vi "Chirp signal generator.vi"(2 "Time per integer frequency [sec]":i32=2, 4 "Append deceleration profile":bool=TRUE, 5 "Amplitude [deg]":dbl, 6 "Error In":errorcluster, 7 "Signal sampling period [ms]":i32=5 step=1, 8 "End frequency \n[Hz, cycles/sec]":i32=10 step=1, 9 "Start frequency \n[Hz, cycles/sec]":i32=1 step=1) -> (0 "error out":errorcluster, 1 "Duration of full profile [sec]":i32, 3 "Full chirp profile":dbl[](array[numeric]))   [LabVIEW 2018]
uses:
  <vilib>/Analysis/NI_AALBase.lvlib
panel:
  out "Sampled deceleration profile":dbl[](array[numeric])
  out "Deceleration profile":cluster{i32, dbl[unit], "Chirp Pattern":dbl[]}(graph)
  out "Samples in full profile":i32
  out "Full chirp profile":T1(graph)={0.0, 0.01, "arbitrary wave"=[]}
  out "Sampled chirp signal":dbl[](array[numeric])
  out "Number of samples in chirp":i32
  out "Chirp duration [sec]":i32
  out "Signal sampling rate \n[Hz, samples/sec]":dbl=100.0 step=1.0 format="%#.3g"
  out "Chirp signal":T2(graph)
  # "INPUTS"
  # "OUTPUTS"
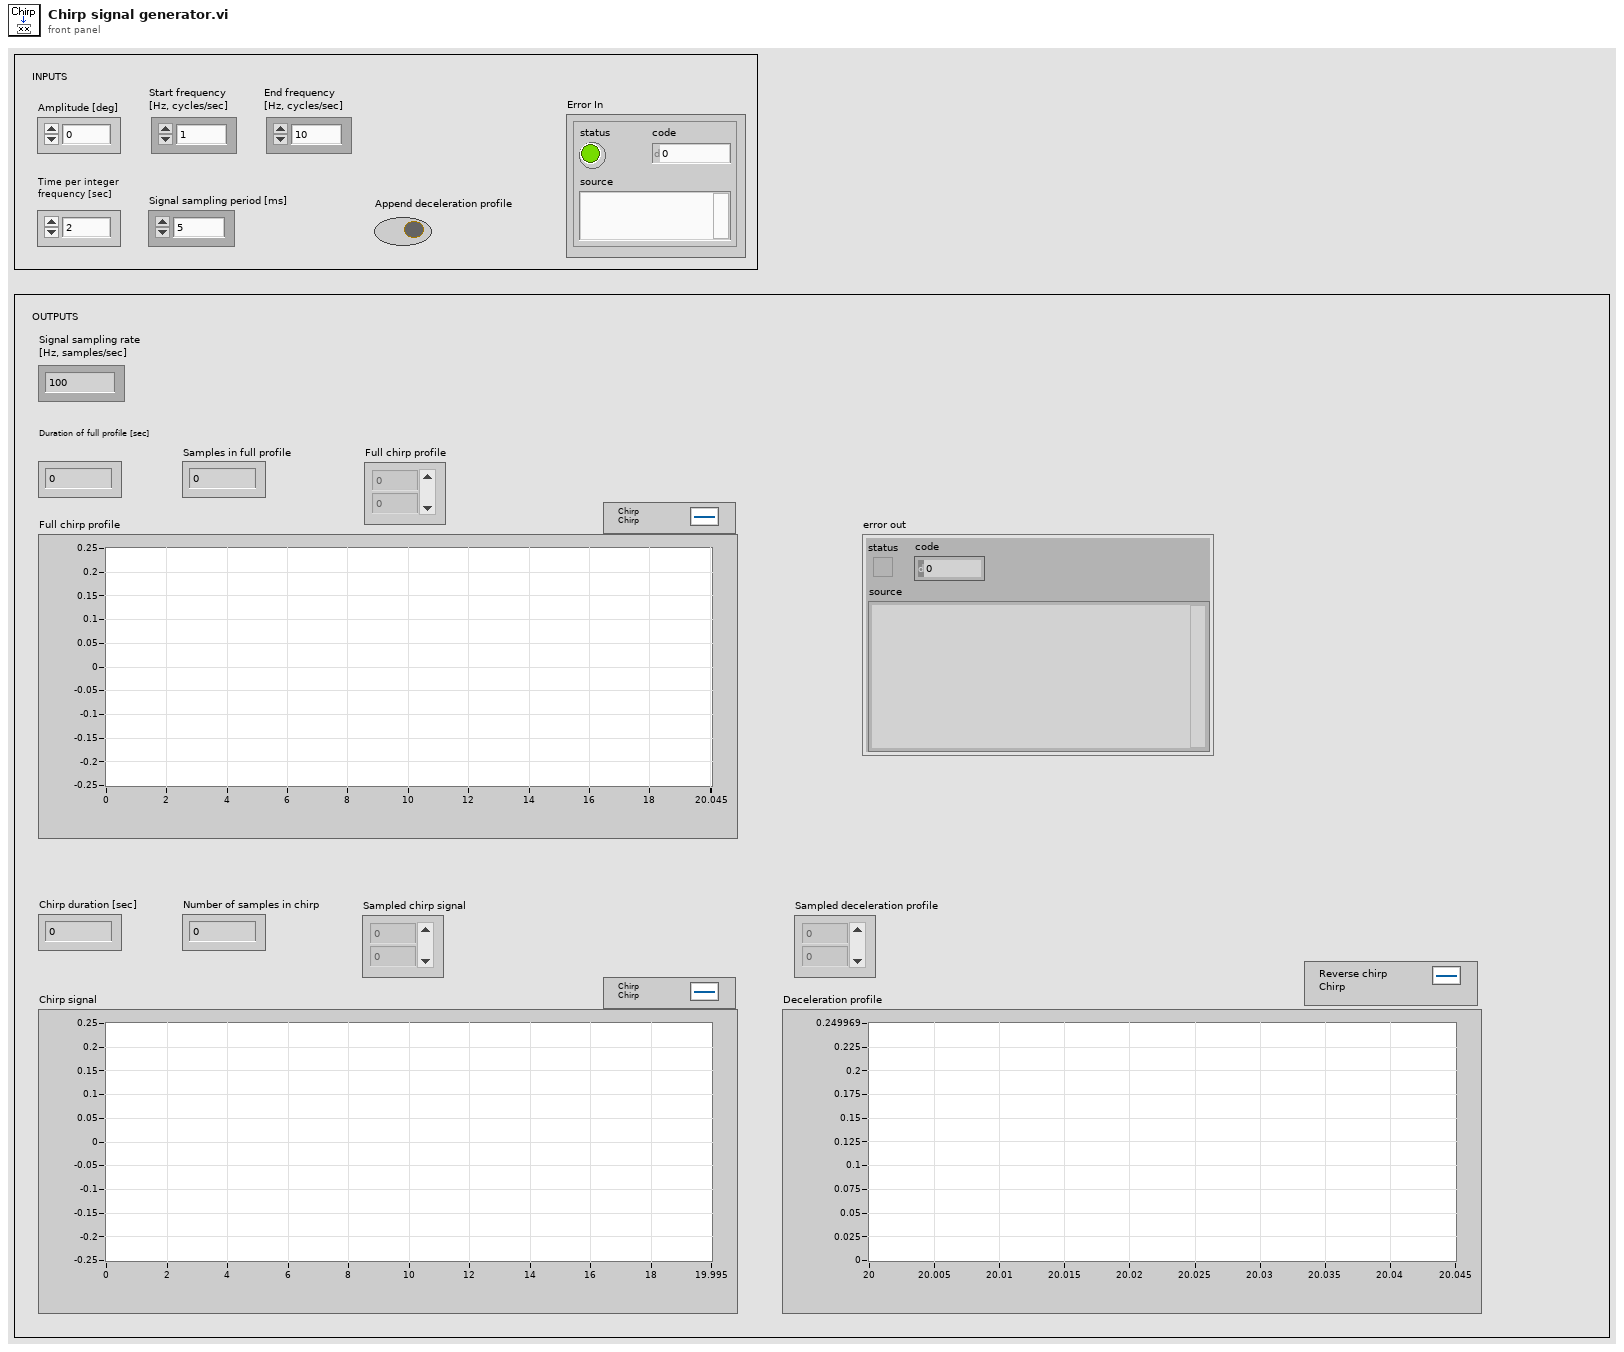
[diagram p1: front panel]
types:
  T1 = cluster{dbl[unit], dbl[unit], "arbitrary wave":dbl[]}
  T2 = cluster{dbl[unit], dbl[unit], "Chirp Pattern":dbl[]}
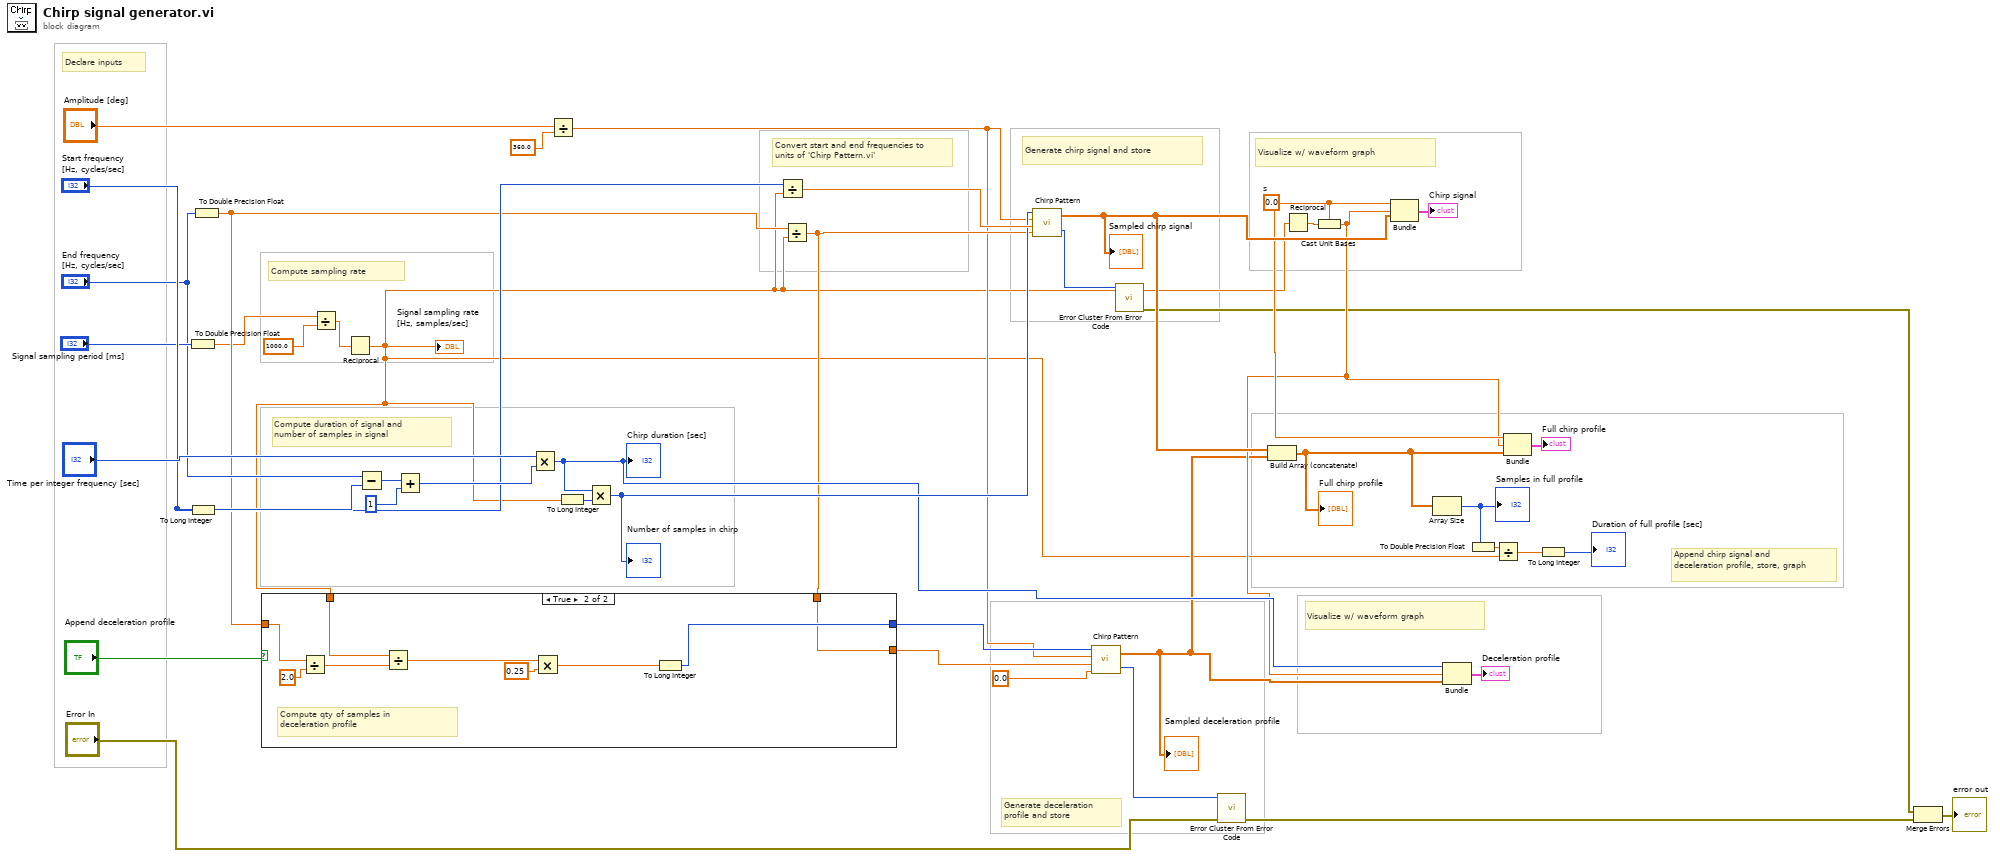
[diagram p0: block diagram]
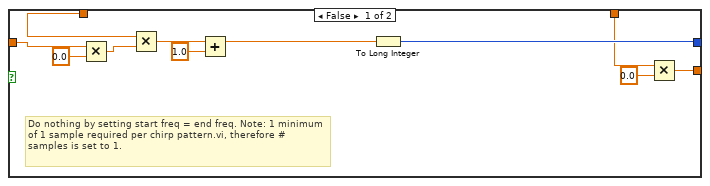
[diagram p2: hidden frame]
diagram:
  w26 = dbl[unit] 0.0  # s
  # "Generate deceleration profile and store"
  # "Visualize w/ waveform graph"
  # "Append chirp signal and deceleration profile, store, graph"
  # "Generate chirp signal and store"
  # "Visualize w/ waveform graph"
  # "Declare inputs"
  # "Convert start and end frequencies to units of 'Chirp Pattern.vi'"
  # "Compute sampling rate"
  # "Compute duration of signal and number of samples in signal"
  n1 = To Double Precision Float(number="Signal sampling period [ms]") -> (double precision float=w8:dbl)
  n2 = To Long Integer(number="Start frequency \n[Hz, cycles/sec]") -> (32bit integer=w33:i32)
  n3 = To Double Precision Float(number="End frequency \n[Hz, cycles/sec]") -> (double precision float=w31:dbl)
  n4 = Divide(x=w8, y=1000.0) -> (x/y=w6:dbl)
  n5 = Reciprocal(x=w6) -> (1/x=w2:dbl)
  "Signal sampling rate \n[Hz, samples/sec]" <- w2
  n6 = Subtract(x="End frequency \n[Hz, cycles/sec]", y="Start frequency \n[Hz, cycles/sec]") -> (x-y=w32:i32)
  n7 = Add(x=w32, y=1) -> (x+y=w44:i32)
  n8 = Multiply(x="Time per integer frequency [sec]", y=w44) -> (x*y=w19:i32)
  "Chirp duration [sec]" <- w19
  n9 = Divide(x="Amplitude [deg]", y=360.0) -> (x/y=w11:dbl)
  n10 = To Long Integer(number=w2) -> (32bit integer=w7:i32)
  n11 = Multiply(x=w19, y=w7) -> (x*y=w37:i32)
  "Number of samples in chirp" <- w37
  n12 = Divide(x=w33, y=w2) -> (x/y=w41:dbl)
  n13 = Divide(x=w31, y=w2) -> (x/y=w14:dbl)
  n14 = case shown="True" "Append deceleration profile" {
    tunnel: w31 -> [w55 w64]
    tunnel: w2 -> [w53 w58]
    tunnel: [w50 w57] -> w20
    tunnel: w14 -> [w47 w56]
    tunnel: [w45 w56] -> w13
    frame False {
      # "Do nothing by setting start freq = end freq. Note: 1 minimum of 1 sample required per chirp pattern.vi, therefore # samples is set to 1."
      n15 = Multiply(x=w55, y=0.0) -> (x*y=w52:dbl)
      n16 = Multiply(x=w53, y=w52) -> (x*y=w51:dbl)
      n17 = Add(x=w51, y=1.0) -> (x+y=w49:dbl)
      n18 = To Long Integer(number=w49) -> (32bit integer=w50:i32)
      n19 = Multiply(x=w47, y=0.0) -> (x*y=w45:dbl)
    }
    frame True {
      # "Compute qty of samples in deceleration profile"
      n20 = Divide(x=w64, y=2.0) -> (x/y=w62:dbl)
      n21 = Divide(x=w58, y=w62) -> (x/y=w61:dbl)
      n22 = Multiply(x=w61, y=0.25) -> (x*y=w59:dbl)
      n23 = To Long Integer(number=w59) -> (32bit integer=w57:i32)
    }
  }
  n24 = call <vilib>:"Chirp Pattern.vi"("f2"=w14, "f1"=w41, "amplitude"=w11, "samples"=w37) -> ("error"=w35:i32, "Chirp Pattern"=w29:dbl[])
  "Sampled chirp signal" <- w29
  n25 = call <vilib>:"Chirp Pattern.vi"("f2"=0.0, "f1"=w13, "amplitude"=w11, "samples"=w20) -> ("error"=w21:i32, "Chirp Pattern"=w15:dbl[])
  "Sampled deceleration profile" <- w15
  n26 = call <vilib>:"Error Cluster From Error Code.vi"("error code (0)"=w35) -> ("error out"=w16:errorcluster)  [unwired: 8 in]
  n27 = call <vilib>:"Error Cluster From Error Code.vi"("error in (no error)"="Error In", "error code (0)"=w21) -> ("error out"=w17:errorcluster)  [unwired: 7 in]
  n28 = Build Array (concatenate)(w29, w15) -> (w25:dbl[])
  "Full chirp profile" <- w25
  n29 = Reciprocal(x=w2) -> (1/x=w40:dbl)
  n30 = Cast Unit Bases(0:w40, 1:w26) -> (2:w18:dbl[unit])
  n31 = Bundle(w26, w18, "Chirp Pattern"=w29) -> (→"Chirp signal":T2)  [unwired: 1 in]
  n32 = Array Size(array=w25) -> (size(s)=w24:i32)
  "Samples in full profile" <- w24
  n33 = Bundle(w19, w18, "Chirp Pattern"=w15) -> (→"Deceleration profile":cluster{i32, dbl[unit], "Chirp Pattern":dbl[]})  [unwired: 1 in]
  n34 = To Double Precision Float(number=w24) -> (double precision float=w1:dbl)
  n35 = Divide(x=w1, y=w2) -> (x/y=w4:dbl)
  n36 = Bundle(w26, w18, w25) -> (→"Full chirp profile":cluster{dbl[unit], dbl[unit], dbl[]})  [unwired: 1 in]
  n37 = To Long Integer(number=w4) -> (32bit integer=→"Duration of full profile [sec]":i32)
  n38 = Merge Errors(w16, w17) -> (→"error out":errorcluster)
